vi "Plot Style Chooser Dialog.vi"(3 "Error In":errorcluster) -> (6 "Plot Style out":T1={"Plot Style"=enum."unchanged", "Histogram Type"=enum."Left Bound", "Line Tickness"=enum."unchanged", "Line Style"=enum."unchanged", "Point Style"=enum."unchanged", "Line Color"=0, "Point Color"=0, "Anti-aliased"=FALSE, "Line Color Chooser"=enum."unchanged", "Point Color Chooser"=enum."unchanged", "Line Color List"="", "Point Color List"=""}, 7 "Cancelled?":bool, 9 "Error Out":errorcluster)   [LabVIEW 2021, in "Graphs.lvlib"]
uses:
  Graphs.lvlib
  Plot Style 3.ctl
  <vilib>/measure/NI_MABase.lvlib
panel:
  in  "Cancel":bool
  in  "OK":bool
  out "Preview":waveform(dbl)(graph)
  in  "Plot Style":T1={"Plot Style"=enum."unchanged", "Histogram Type"=enum."Left Bound", "Line Tickness"=enum."unchanged", "Line Style"=enum."unchanged", "Point Style"=enum."unchanged", "Line Color"=0, "Point Color"=0, "Anti-aliased"=FALSE, "Line Color Chooser"=enum."unchanged", "Point Color Chooser"=enum."unchanged", "Line Color List"="", "Point Color List"=""}
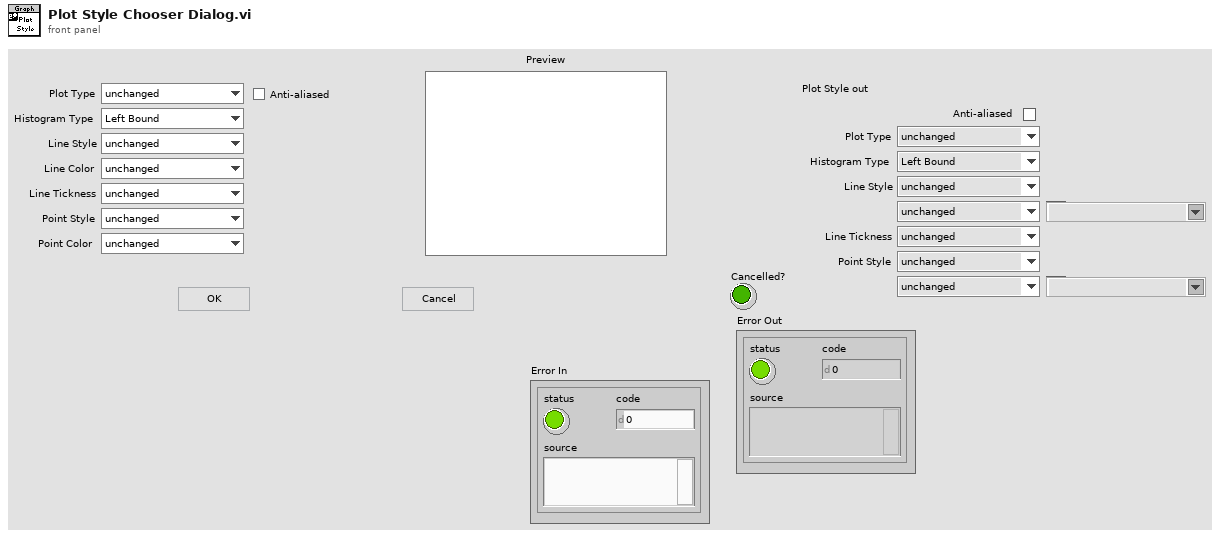
[diagram p1: front panel]
types:
  T1 = typedef "Graphs.lvlib/Plot Style 3.ctl" = cluster{"Plot Style":enum16{"unchanged", "Line", "Symbol", "Line + Symbol", "Histogram", "Histogram + Symbol"}, "Histogram Type":enum16{"unchanged", "Left Bound", "Center", "Right Bound"}, "Line Tickness":enum16{"unchanged", "Thin", "1 pixel", "2 pixel", "3 pixel", "4 pixel", "5 pixel"}, "Line Style":enum16{"unchanged", "Plain", "Long Dash", "Short Dash", "Long-Short Dash", "Long-Short-Short Dash"}, "Point Style":enum16{"unchanged", "None", "Empty Circle", "Filled Circle", "Thick Circle", "Dotted Circle", "Empty Square", "Filled Square", "Thick Square", "Dotted Square", "Small Filled Square", "Dot", "Cross", "Tiny Cross", "Large X", "Small x", "Diamond", "Small Empty Square"}, "Line Color":u32, "Point Color":u32, "Anti-aliased":bool, "Line Color Chooser":enum16{"unchanged", "Color Box", "Color List"}, "Point Color Chooser":enum16{"unchanged", "Color Box", "Color List"}, "Line Color List":string, "Point Color List":string}
  T2 = enum16{"Sine Wave", "Triangle Wave", "Square Wave", "Sawtooth Wave"}
  T3 = typedef "Graphs.lvlib/Single Plot Style 2.ctl" = cluster{"Plot Style":enum16{"unchanged", "Line", "Symbol", "Line + Symbol", "Histogram", "Histogram + Symbol"}, "Histogram Type":enum16{"unchanged", "Left Bound", "Center", "Right Bound"}, "Line Tickness":enum16{"unchanged", "Thin", "1 pixel", "2 pixel", "3 pixel", "4 pixel", "5 pixel"}, "Line Style":enum16{"unchanged", "Plain", "Long Dash", "Short Dash", "Long-Short Dash", "Long-Short-Short Dash"}, "Point Style":enum16{"unchanged", "None", "Empty Circle", "Filled Circle", "Thick Circle", "Dotted Circle", "Empty Square", "Filled Square", "Thick Square", "Dotted Square", "Small Filled Square", "Dot", "Cross", "Tiny Cross", "Large X", "Small x", "Diamond", "Small Empty Square"}, "Line Color":u32, "Line Color defined?":bool, "Point Color":u32, "Point Color defined?":bool, "Anti-aliased":bool}
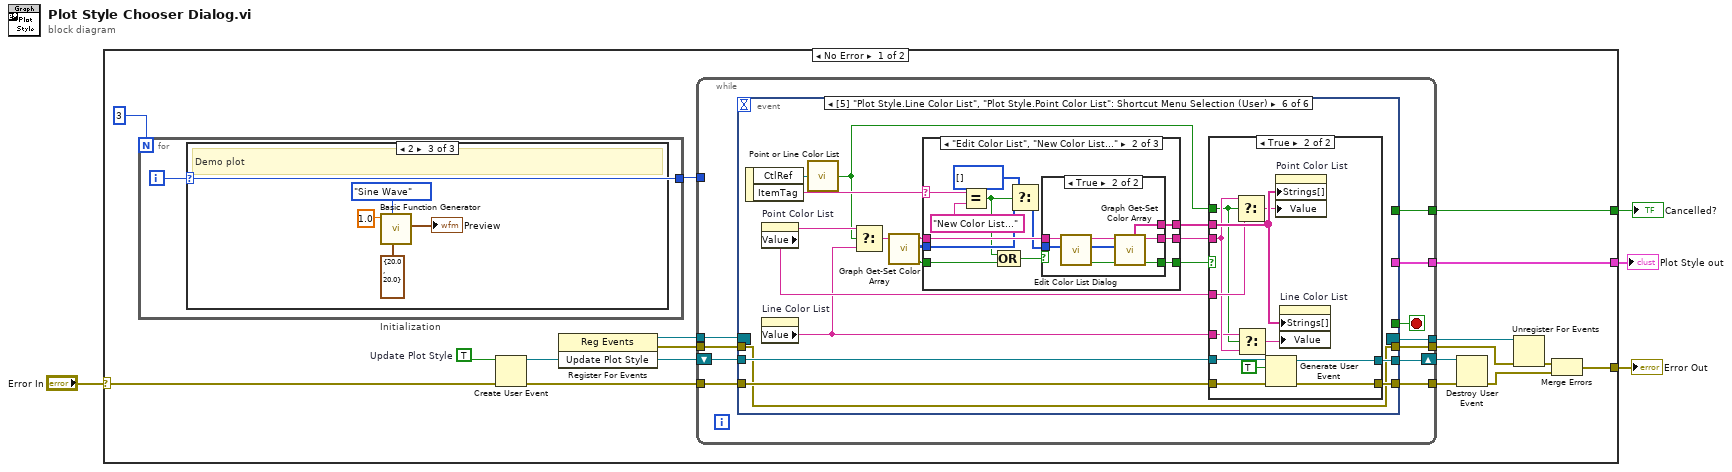
[diagram p0: block diagram]
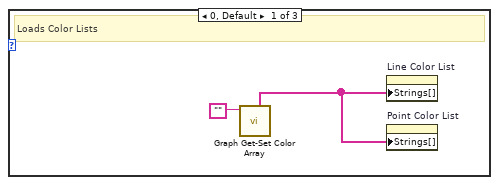
[diagram p2: hidden frame]
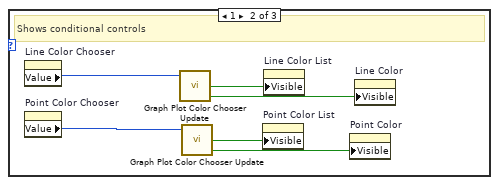
[diagram p3: hidden frame]
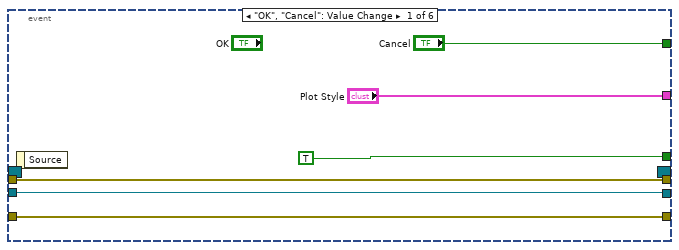
[diagram p4: hidden frame]
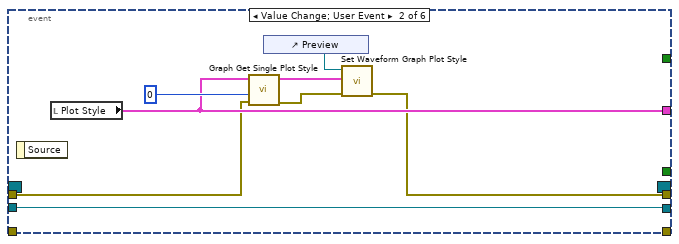
[diagram p5: hidden frame]
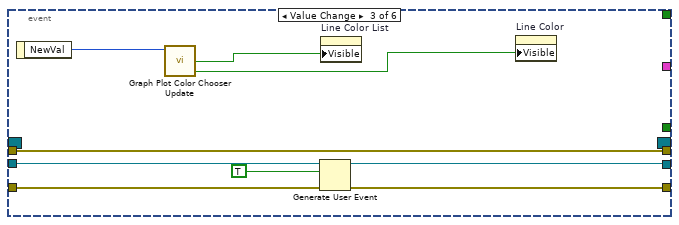
[diagram p6: hidden frame]
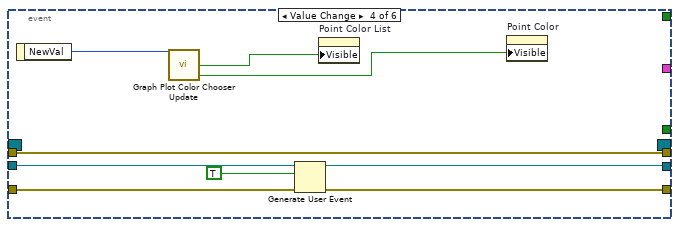
[diagram p7: hidden frame]
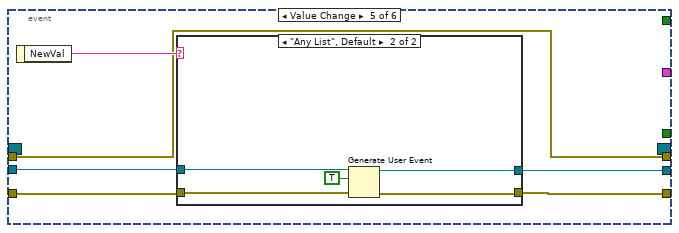
[diagram p8: hidden frame]
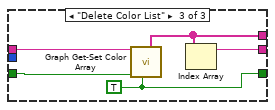
[diagram p13: hidden frame]
diagram:
  n1 = case shown="No Error" "Error In" {
    selector: "Error In" -> [w12 w147]
    tunnel: [w6 w147] -> w3
    tunnel: [w14 _] -> w2
    tunnel: [w13 _] -> w1
    frame No Error {
      w19 = TRUE  # Update Plot Style
      n2 = for "Initialization" {
        N: 3 -> [_]
        tunnel: [w22] -> w20
        i -> [w22]
        n3 = case shown="2" w22 {
          frame 0, Default {
            # "Loads Color Lists"
            n4 = call "Graph Get-Set Color Array.vi"("Color List Name"="") -> ("[Color List Name]"=w24:string[])  [unwired: 5 in, 5 out]
            n5 = property on="Line Color List" class="CmbBox"("Strings[]"=w24) -> ()  [unwired: 2 in, 2 out]
            n6 = property on="Point Color List" class="CmbBox"("Strings[]"=w24) -> ()  [unwired: 2 in, 2 out]
          }
          frame 1 {
            # "Shows conditional controls"
            n7 = property on="Line Color Chooser" class="Enum (strict)"() -> ("Value"=w27:enum16{"unchanged", "Color Box", "Color List"})  [unwired: 2 in, 2 out]
            n8 = property on="Point Color Chooser" class="Enum (strict)"() -> ("Value"=w30:enum16{"unchanged", "Color Box", "Color List"})  [unwired: 2 in, 2 out]
            n9 = call "Graph Plot Color Chooser Update.vi"("Color Chooser"=w27) -> ("Color Box Visible"=w25:bool, "Color List Visible"=w26:bool)  [unwired: 3 in]
            n10 = call "Graph Plot Color Chooser Update.vi"("Color Chooser"=w30) -> ("Color Box Visible"=w28:bool, "Color List Visible"=w29:bool)  [unwired: 3 in]
            n11 = property on="Point Color List" class="CmbBox"("Visible"=w29) -> ()  [unwired: 2 in, 2 out]
            n12 = property on="Line Color List" class="CmbBox"("Visible"=w26) -> ()  [unwired: 2 in, 2 out]
            n13 = property on="Point Color" class="ColBox"("Visible"=w28) -> ()  [unwired: 2 in, 2 out]
            n14 = property on="Line Color" class="ColBox"("Visible"=w25) -> ()  [unwired: 2 in, 2 out]
          }
          frame 2 {
            # "Demo plot"
            n15 = call <vilib>:"Basic Function Generator.vi"("sampling info"=cluster{"Fs":dbl, "#s":dbl} {"Fs"=20.0, "#s"=20.0}, "signal type"=T2."Sine Wave", "frequency"=1.0) -> ("signal out"=→"Preview":waveform(dbl))  [unwired: 6 in, 2 out]
          }
        }
      }
      n16 = Create User Event(user event datatype=w19, error in=w12) -> (user event=w16:refnum<user-event>, error out=w8:errorcluster)
      n17 = register-events(w16) -> (reference out=w18:refnum<event-registration>, error out=w11:errorcluster)  [unwired: 2 in]
      n18 = while {
        tunnel: [w44] -> w13
        tunnel: [w43] -> w14
        tunnel: w20 -> [_]
        tunnel: w18 -> [w42]
        tunnel: [w41] -> w17
        shift-right: [w39] -> w15
        shift-left: w16 -> [w40]
        tunnel: w11 -> [w38]
        tunnel: [w37] -> w9
        tunnel: w8 -> [w36]
        tunnel: [w35] -> w7
        stop <- w45 stop-if-true
        n19 = event shown="[5] \"Plot Style.Line Color List\", \"Plot Style.Point Color List\": Shortcut Menu Selection (User)" {
          selector: w42 -> [_ _ _ _ _ _]
          dyn-events: [_ _ _ _ _ _] -> w41
          timeout: _ -> [_ _ _ _ _ _]
          tunnel: [TRUE _ _ _ _ _] -> w45
          tunnel: ["Plot Style" w54 _ _ _ _] -> w44
          tunnel: ["Cancel" _ _ _ _ _] -> w43
          tunnel: w40 -> [w49 w55 w68 w77 w82 w101]
          tunnel: [w49 w55 w67 w76 w81 w100] -> w39
          tunnel: w38 -> [w46 w53 w60 w69 w78 w92]
          tunnel: [w47 _ w62 w70 w79 w93] -> w37
          tunnel: w36 -> [w47 _ w61 w71 w80 w94]
          tunnel: [w46 w52 w60 w69 w78 w92] -> w35
          event "OK", "Cancel": Value Change {
            n20 = event-data() -> ()  [unwired: 1 in, 1 out]
          }
          event Value Change; User Event {
            n21 = event-data() -> ()  [unwired: 1 in, 1 out]
            n22 = local read "Plot Style"() -> (w54:T1)
            n23 = call "Graph Get Single Plot Style.vi"("Error In"=w53, "index"=0, "Plot Style in"=w54) -> ("Error Out"=w56:errorcluster, "Plot Style out"=w58:T3)  [unwired: 7 in]
            n24 = control-ref of="Preview"() -> (w59:refnum<vi>)
            n25 = call "Set Waveform Graph Plot Style.vi"("Error In"=w56, "Plot Style"=w58, "Graph in"=w59) -> ("Error Out"=w52:errorcluster)  [unwired: 8 in]
          }
          event Value Change {
            n26 = event-data() -> ("NewVal"=w65:enum16{"unchanged", "Color Box", "Color List"})  [unwired: 1 in]
            n27 = call "Graph Plot Color Chooser Update.vi"("Color Chooser"=w65) -> ("Color Box Visible"=w63:bool, "Color List Visible"=w64:bool)  [unwired: 3 in]
            n28 = Generate User Event(user event=w68, event data cluster=TRUE ("event data"), error in=w61) -> (user event out=w67:refnum<user-event>, error out=w62:errorcluster)  [unwired: 1 in]
            n29 = property on="Line Color List" class="CmbBox"("Visible"=w64) -> ()  [unwired: 2 in, 2 out]
            n30 = property on="Line Color" class="ColBox"("Visible"=w63) -> ()  [unwired: 2 in, 2 out]
          }
          event Value Change {
            n31 = event-data() -> ("NewVal"=w74:enum16{"unchanged", "Color Box", "Color List"})  [unwired: 1 in]
            n32 = call "Graph Plot Color Chooser Update.vi"("Color Chooser"=w74) -> ("Color Box Visible"=w72:bool, "Color List Visible"=w73:bool)  [unwired: 3 in]
            n33 = Generate User Event(user event=w77, event data cluster=TRUE ("event data"), error in=w71) -> (user event out=w76:refnum<user-event>, error out=w70:errorcluster)  [unwired: 1 in]
            n34 = property on="Point Color List" class="CmbBox"("Visible"=w73) -> ()  [unwired: 2 in, 2 out]
            n35 = property on="Point Color" class="ColBox"("Visible"=w72) -> ()  [unwired: 2 in, 2 out]
          }
          event Value Change {
            n36 = event-data() -> ("NewVal"=w83:string)  [unwired: 1 in]
            n37 = case shown="\"Any List\", Default" w83 {
              tunnel: w82 -> [w85 w90]
              tunnel: [w85 w88] -> w81
              tunnel: w80 -> [w84 w87]
              tunnel: [w84 w86] -> w79
              frame "" {
              }
              frame "Any List", Default {
                n38 = Generate User Event(user event=w90, event data cluster=TRUE ("event data"), error in=w87) -> (user event out=w88:refnum<user-event>, error out=w86:errorcluster)  [unwired: 1 in]
              }
            }
          }
          event Shortcut Menu Selection (User) {
            n39 = event-data() -> ("CtlRef"=w99:refnum<vi>, "ItemTag"=w107:string)  [unwired: 1 in]
            n40 = property on="Point Color List" class="CmbBox"() -> ("Value"=w96:string)  [unwired: 2 in, 2 out]
            n41 = property on="Line Color List" class="CmbBox"() -> ("Value"=w95:string)  [unwired: 2 in, 2 out]
            n42 = call "Point or Line Color List.vi"("Color List"=w99) -> ("Point (T)/ Line (F)"=w91:bool)  [unwired: 8 in]
            n43 = Select(t=w96, s=w91, f=w95) -> (s? t:f=w98:string)
            n44 = call "Graph Get-Set Color Array.vi"("Color List Name"=w98) -> ("Found?"=w104:bool, "Color Array out"=w105:u32[], "Color List Name dup"=w106:string)  [unwired: 5 in, 3 out]
            n45 = case shown="\"Edit Color List\", \"New Color List...\"" w107 {
              selector: w107 -> [_ w130 _]
              tunnel: w106 -> [_ w128 w146]
              tunnel: w105 -> [_ w127 _]
              tunnel: w104 -> [_ w133 w145]
              tunnel: [_ w132 w142] -> w103
              tunnel: [_ w131 w144] -> w102
              tunnel: [_ w122 w143] -> w97
              frame "", Default {
              }
              frame "Edit Color List", "New Color List..." {
                n46 = Equal?(x=w130, y="New Color List...") -> (x = y?=w123:bool)
                n47 = Compound Arithmetic op=OR(w123, w133) -> (w124:bool)
                n48 = Select(t=u32[] [], s=w123, f=w127) -> (s? t:f=w125:u32[])
                n49 = case shown="True" w124 {
                  tunnel: w128 -> [_ w141]
                  tunnel: w125 -> [_ w140]
                  tunnel: [_ w136] -> w132
                  tunnel: [_ w135] -> w131
                  tunnel: [_ w134] -> w122
                  frame False {
                  }
                  frame True {
                    n50 = call "Edit Color List Dialog.vi"("Color List"=w140, "Color List Name"=w141) -> ("OK?"=w137:bool, "Color List (out)"=w138:u32[], "Color List Name (out)"=w139:string)  [unwired: 7 in]
                    n51 = call "Graph Get-Set Color Array.vi"("Get (F)/Set"=w137, "Color Array in"=w138, "Color List Name"=w139) -> ("Found?"=w136:bool, "Color List Name dup"=w134:string, "[Color List Name]"=w135:string[])  [unwired: 3 in, 3 out]
                  }
                }
              }
              frame "Delete Color List" {
                w142 = TRUE ("Clear All (F)")
                n52 = call "Graph Get-Set Color Array.vi"("Clear All (F)"=w142, "Get (F)/Set"=w145, "Color List Name"=w146) -> ("[Color List Name]"=w144:string[])  [unwired: 3 in, 5 out]
                n53 = Index Array(array=w144) -> (element=w143:string)  [unwired: 1 in]
              }
            }
            n54 = case shown="True" w103 {
              tunnel: w102 -> [_ w121]
              tunnel: w101 -> [w109 w120]
              tunnel: [w109 w119] -> w100
              tunnel: w91 -> [_ w112]
              tunnel: w97 -> [_ w114]
              tunnel: w96 -> [_ w116]
              tunnel: w95 -> [_ w113]
              tunnel: w94 -> [w108 w111]
              tunnel: [w108 w110] -> w93
              frame False {
              }
              frame True {
                n55 = Select(t=w114, s=w112, f=w116) -> (s? t:f=w117:string)
                n56 = Select(t=w113, s=w112, f=w114) -> (s? t:f=w115:string)
                n57 = Generate User Event(user event=w120, event data cluster=TRUE ("event data"), error in=w111) -> (user event out=w119:refnum<user-event>, error out=w110:errorcluster)  [unwired: 1 in]
                n58 = property on="Point Color List" class="CmbBox"("Strings[]"=w121, "Value"=w117) -> ()  [unwired: 2 in, 2 out]
                n59 = property on="Line Color List" class="CmbBox"("Strings[]"=w121, "Value"=w115) -> ()  [unwired: 2 in, 2 out]
              }
            }
          }
        }
      }
      n60 = Destroy User Event(user event=w15, error in=w9) -> (error out=w5:errorcluster)
      n61 = Unregister For Events(event registration refnum=w17, error in=w7) -> (error out=w10:errorcluster)
      n62 = Merge Errors(w10, w5) -> (w6:errorcluster)
    }
    frame Error {
    }
  }
  "Error Out" <- w3
  "Cancelled?" <- w2
  "Plot Style out" <- w1
